vi "Module Angle Offset (SubVI).vi"(10 "angleOffset":dbl, 11 "absoluteAngle":dbl) -> (3 "absoluteAngle":dbl)   [LabVIEW 2020]
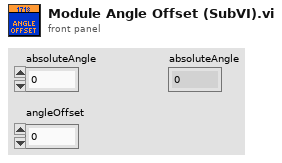
[diagram p1: front panel]
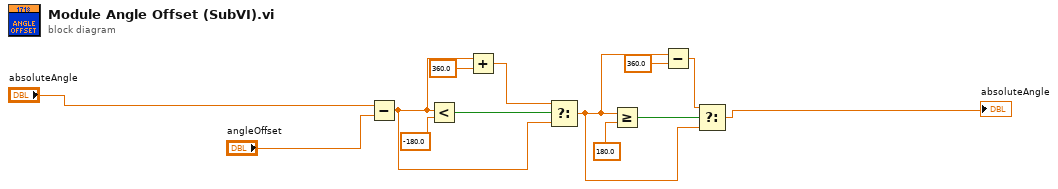
[diagram p0: block diagram]
diagram:
  n1 = Subtract(x="absoluteAngle", y="angleOffset") -> (x-y=w13:dbl)
  n2 = Less?(x=w13, y=-180.0) -> (x < y?=w10:bool)
  n3 = Add(x=w13, y=360.0) -> (x+y=w12:dbl)
  n4 = Select(t=w12, s=w10, f=w13) -> (s? t:f=w2:dbl)
  n5 = Greater Or Equal?(x=w2, y=180.0) -> (x >= y?=w5:bool)
  n6 = Subtract(x=w2, y=360.0) -> (x-y=w3:dbl)
  n7 = Select(t=w3, s=w5, f=w2) -> (s? t:f=→"absoluteAngle":dbl)
